vi "Calibrate Ticks 2 Button Speed (uSMC).vi"(1 "Ticks":u16) -> (0 "Speed (Full Steps/Sec)":u16)   [LabVIEW 2010, in "SignalWriterMH110203USBStepperMotor.lvclass"]
uses:
  SignalWriterMH110203USBStepperMotor.lvclass
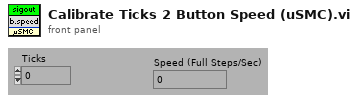
[diagram p1: front panel]
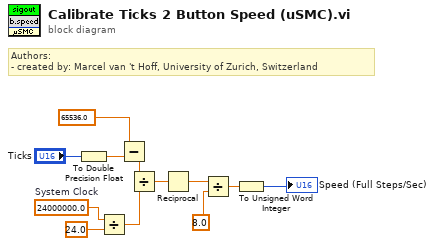
[diagram p0: block diagram]
diagram:
  w12 = 24000000.0  # System Clock
  # "Authors: \n- created by: Marcel van 't Hoff, University of Zurich, Switzerland"
  n1 = To Double Precision Float(number="Ticks") -> (double precision float=w8:dbl)
  n2 = Divide(x=w12, y=24.0) -> (x/y=w7:dbl)
  n3 = Subtract(x=65536.0, y=w8) -> (x-y=w2:dbl)
  n4 = Divide(x=w2, y=w7) -> (x/y=w6:dbl)
  n5 = Reciprocal(x=w6) -> (1/x=w1:dbl)
  n6 = Divide(x=w1, y=8.0) -> (x/y=w4:dbl)
  n7 = To Unsigned Word Integer(number=w4) -> (unsigned 16bit integer=→"Speed (Full Steps/Sec)":u16)
